vi "Tach Get Missing Pulses.vi"(11 "pulse positions":dbl[](array[numeric]) format="%.2f") -> (2 "pulses inserted":i32, 3 "modified pulse positions":dbl[](array[numeric]) format="%.2f")   [LabVIEW 2017, in "VibrationAnalysisFunctions.lvlib"]
uses:
  <vilib>/addons/InsightCM/Utilities/Analysis/Vibration/VibrationAnalysisFunctions.lvlib
  <vilib>/Analysis/NI_AALBase.lvlib
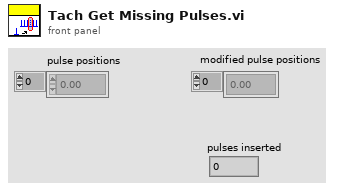
[diagram p1: front panel]
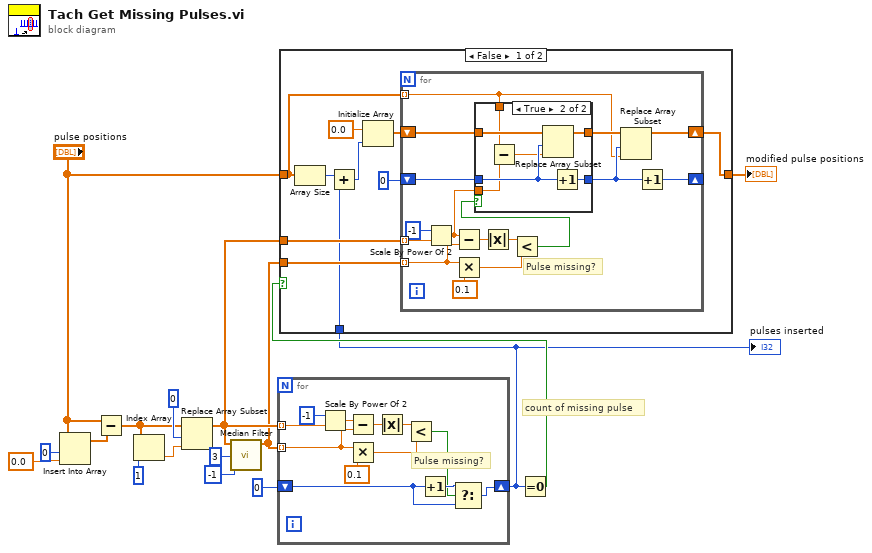
[diagram p0: block diagram]
diagram:
  # "count of missing pulse"
  n1 = Insert Into Array(array="pulse positions", index=0 ("Index"), new element=0.0) -> (w5:dbl[])
  n2 = Subtract(x="pulse positions", y=w5) -> (x-y=w3:dbl[])
  n3 = Index Array(array=w3, index=1 ("Index")) -> (element=w15:dbl)
  n4 = Replace Array Subset(array=w3, new element=w15, index=0 ("Index")) -> (w10:dbl[])
  n5 = call <vilib>:"Median Filter.vi"("right rank"=-1, "left rank"=3, "X"=w10) -> ("Filtered X"=w9:dbl[])  [unwired: 7 in, 1 out]
  n6 = for {
    tunnel: w10 -> [w17] mode=indexing
    tunnel: w9 -> [w18] mode=indexing
    shift-right: [w28] -> w8
    shift-left: 0 -> [w26]
    # "Pulse missing?"
    n7 = Scale By Power Of 2(n=-1, x=w17) -> (x*2^n=w20:dbl)
    n8 = Subtract(x=w20, y=w18) -> (x-y=w25:dbl)
    n9 = Multiply(x=w18, y=0.1) -> (x*y=w22:dbl)
    n10 = Absolute Value(x=w25) -> (abs(x)=w24:dbl)
    n11 = Less?(x=w24, y=w22) -> (x < y?=w19:bool)
    n12 = Increment(x=w26) -> (x+1=w27:i32)
    n13 = Select(t=w27, s=w19, f=w26) -> (s? t:f=w28:i32)
  }
  "pulses inserted" <- w8
  n14 = Equal To 0?(x=w8) -> (x = 0?=w11:bool)
  n15 = case shown="False" w11 {
    tunnel: "pulse positions" -> [w30 w64]
    tunnel: [w31 w64] -> w12
    tunnel: w10 -> [w35 _]
    tunnel: w9 -> [w34 _]
    tunnel: w8 -> [w29 _]
    frame False {
      n16 = Array Size(array=w30) -> (size(s)=w37:i32)
      n17 = Add(x=w37, y=w29) -> (x+y=w36:i32)
      n18 = Initialize Array(0.0 ("Element Data"), w36) -> (w33:dbl[])
      n19 = for {
        tunnel: w35 -> [w47] mode=indexing
        tunnel: w34 -> [w46] mode=indexing
        shift-right: [w41] -> w31
        shift-left: w33 -> [w44]
        shift-right: [w43] -> _
        shift-left: 0 -> [w49]
        tunnel: w30 -> [w39] mode=indexing
        # "Pulse missing?"
        n20 = Scale By Power Of 2(n=-1, x=w47) -> (x*2^n=w45:dbl)
        n21 = Subtract(x=w45, y=w46) -> (x-y=w54:dbl)
        n22 = Multiply(x=w46, y=0.1) -> (x*y=w51:dbl)
        n23 = Absolute Value(x=w54) -> (abs(x)=w53:dbl)
        n24 = Less?(x=w53, y=w51) -> (x < y?=w50:bool)
        n25 = case shown="True" w50 {
          tunnel: [w56 w61] -> w42
          tunnel: w44 -> [w56 w62]
          tunnel: w49 -> [w55 w60]
          tunnel: [w55 w63] -> w40
          tunnel: w39 -> [_ w59]
          tunnel: w45 -> [_ w57]
          frame False {
          }
          frame True {
            n26 = Subtract(x=w59, y=w57) -> (x-y=w58:dbl)
            n27 = Replace Array Subset(array=w62, new element=w58, index=w60) -> (w61:dbl[])
            n28 = Increment(x=w60) -> (x+1=w63:i32)
          }
        }
        n29 = Replace Array Subset(array=w42, new element=w39, index=w40) -> (w41:dbl[])
        n30 = Increment(x=w40) -> (x+1=w43:i32)
      }
    }
    frame True {
    }
  }
  "modified pulse positions" <- w12
